vi "Initialize Kinect.vi"(8 "error in (no error)":errorcluster, 11 "Buffer Size":i32=1) -> (0 "error out":errorcluster, 2 "Queues Out":T1, 3 "References":T2)   [LabVIEW 2010, in "Kinect_API.lvlib"]
uses:
  Kinect_API.lvlib
  Microsoft.Research.Kinect
  <vilib>/vision/Image Controls.llb/IMAQ Image.ctl
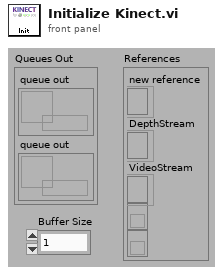
[diagram p1: front panel]
types:
  T1 = cluster{"queue out":refnum<queue>, "queue out":refnum<queue>}
  T2 = cluster{"new reference":refnum<k24>, "DepthStream":refnum<k24>, "VideoStream":refnum<k24>, "Event Callback":refnum<k27>, "Event Callback":refnum<k27>}
  T3 = typedef "IMAQ Image.ctl" = refnum<image>
  T4 = cluster{"new reference":refnum<k24>, "DepthStream":refnum<k24>, "VideoStream":refnum<k24>, refnum<k27>, refnum<k27>}
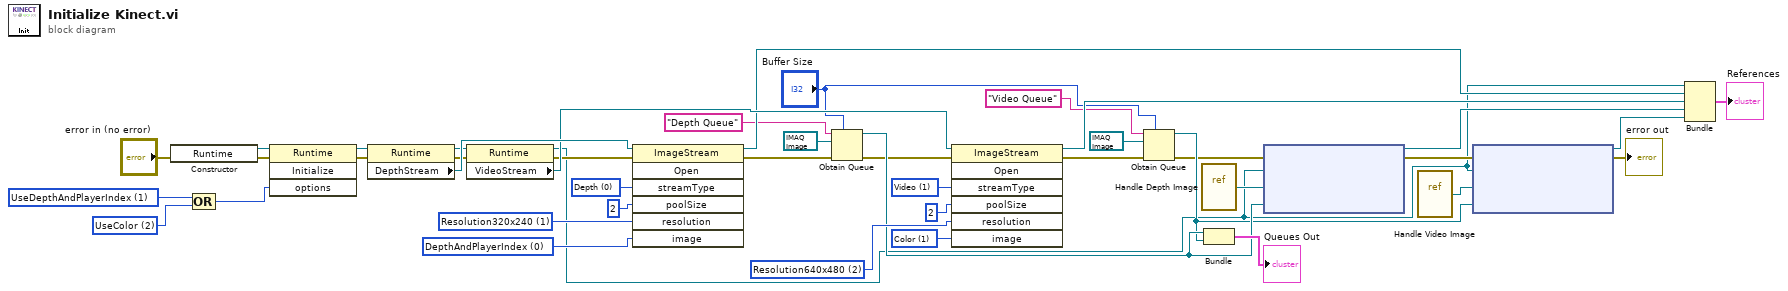
[diagram p0: block diagram]
diagram:
  w25 = 2 items=["UseDepthAndPlayerIndex"=1, "UseColor"=2, "UseSkeletalTracking"=8, "UseDepth"=32] ("options")
  w35 = 1 items=["Resolution80x60"=0, "Resolution320x240"=1, "Resolution640x480"=2, "Resolution1280x1024"=3, "Invalid"=-1] ("resolution")
  w26 = 1 items=["UseDepthAndPlayerIndex"=1, "UseColor"=2, "UseSkeletalTracking"=8, "UseDepth"=32] ("options")
  w38 = 0 items=["DepthAndPlayerIndex", "Color", "ColorYuv", "ColorYuvRaw", "Depth", "DepthAndPlayerIndexInColorSpace", "DepthInColorSpace", "ColorInDepthSpace"] ("image")
  w30 = 1 items=["DepthAndPlayerIndex", "Color", "ColorYuv", "ColorYuvRaw", "Depth", "DepthAndPlayerIndexInColorSpace", "DepthInColorSpace", "ColorInDepthSpace"] ("image")
  w31 = 2 items=["Resolution80x60"=0, "Resolution320x240"=1, "Resolution640x480"=2, "Resolution1280x1024"=3, "Invalid"=-1] ("resolution")
  w33 = 1 items=["Depth"=0, "Video"=1, "Invalid"=-1] ("streamType")
  w41 = 0 items=["Depth"=0, "Video"=1, "Invalid"=-1] ("streamType")
  n1 = constructor class="Runtime"(error in="error in (no error)") -> (reference out=w39:refnum<k24>, error out=w37:errorcluster)  [unwired: 2 in, 1 out]
  n2 = Compound Arithmetic op=OR(w26, w25) -> (w36:i32)
  n3 = invoke class="Runtime" method="Initialize"(reference=w39, error in=w37, "options"=w36) -> (reference out=w29:refnum<k24>, error out=w43:errorcluster)  [unwired: 1 in, 2 out]
  n4 = property class="Runtime"(reference=w29, error in=w43) -> (reference out=w2:refnum<k24>, error out=w28:errorcluster, "DepthStream"=w42:refnum<k24>)
  n5 = property class="Runtime"(reference=w2, error in=w28) -> (reference out=w1:refnum<k24>, error out=w27:errorcluster, "VideoStream"=w34:refnum<k24>)
  n6 = invoke class="ImageStream" method="Open"(reference=w42, error in=w27, "streamType"=w41, "poolSize"=2, "resolution"=w35, "image"=w38) -> (reference out=w24:refnum<k24>, error out=w6:errorcluster)  [unwired: 1 in, 5 out]
  n7 = Obtain Queue(max queue size (-1, unlimited)="Buffer Size", name (unnamed)="Depth Queue", element data type=T3 refnum ("New Image"), error in (no error)=w6) -> (queue out=w11:refnum<queue>, error out=w5:errorcluster)  [unwired: 1 in, 1 out]
  n8 = invoke class="ImageStream" method="Open"(reference=w34, error in=w5, "streamType"=w33, "poolSize"=2, "resolution"=w31, "image"=w30) -> (reference out=w23:refnum<k24>, error out=w4:errorcluster)  [unwired: 1 in, 5 out]
  n9 = Obtain Queue(max queue size (-1, unlimited)="Buffer Size", name (unnamed)="Video Queue", element data type=T3 refnum ("New Image"), error in (no error)=w4) -> (queue out=w10:refnum<queue>, error out=w3:errorcluster)  [unwired: 1 in, 1 out]
  n10 = vi-ref "Handle Depth Image.vi"() -> ("vi reference"=w9:refnum<vi>)
  n11 = Bundle("queue out"=w11, "queue out"=w10) -> (→"Queues Out":T1)  [unwired: 1 in]
  n12 = node(w3, w1, w9, w11) -> (w22:refnum<k27>, w12:errorcluster)  [unwired: 1 in]
  n13 = vi-ref "Handle Video Image.vi"() -> ("vi reference"=w8:refnum<vi>)
  n14 = node(w12, w1, w8, w10) -> (w21:refnum<k27>, →"error out":errorcluster)  [unwired: 1 in]
  n15 = Bundle("new reference"=w1, "DepthStream"=w24, "VideoStream"=w23, w22, w21) -> (→"References":T4)  [unwired: 1 in]
